vi "validate key value pair.vi"(8 "error in":errorcluster, 9 "value":string, 10 "key":string, 11 "fixed channel configuration in":refnum<class "control module configuration.lvclass">) -> (0 "error out":errorcluster, 3 "fixed channel configuration out":refnum<class "control module configuration.lvclass">)   [LabVIEW 2013, in "control module configuration.lvclass"]
uses:
  control module configuration.lvclass
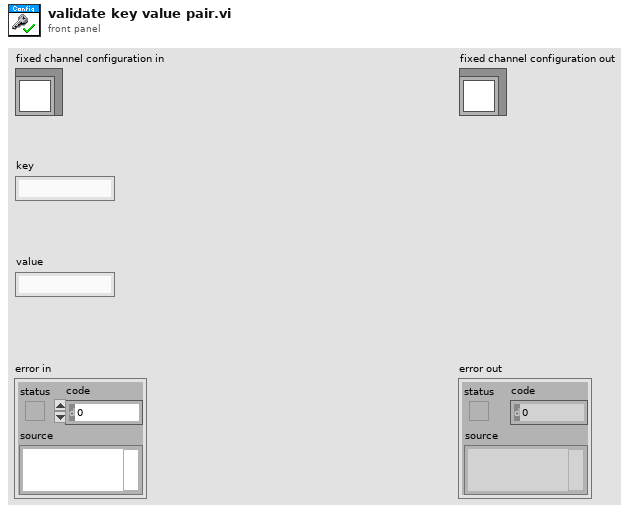
[diagram p1: front panel]
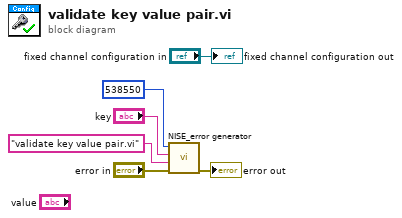
[diagram p0: block diagram]
diagram:
  n1 = call <vilib>:"NISE_error generator.vi"("error in"="error in", "source"="validate key value pair.vi", "append error message"="key", "error code (0)"=538550) -> ("error out"=→"error out":errorcluster)  [unwired: 5 in]
  "fixed channel configuration out" <- "fixed channel configuration in"
